vi "Calibrate_HH.vi"(3 "Deviceindex":i32) -> (0 "Returncode":i32, 1 "Status":string)   [LabVIEW 2009]
uses:
  hhlib.dll
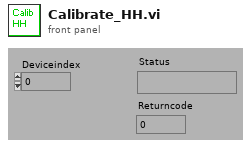
[diagram p1: front panel]
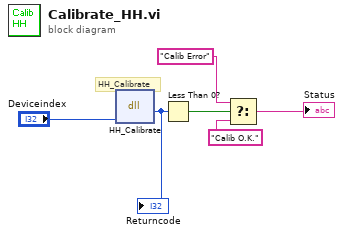
[diagram p0: block diagram]
diagram:
  # "HH_Calibrate"
  n1 = dll-call lib="C:/Programme/Anwendungen/DAQLinescan_HH/hhlib.dll" fn="HH_Calibrate"("devidx"="Deviceindex") -> (w4:i32)  [unwired: 4 in, 2 out]
  "Returncode" <- w4
  n2 = Less Than 0?(x=w4) -> (x < 0?=w2:bool)
  n3 = Select(t="Calib Error", s=w2, f="Calib O.K.") -> (s? t:f=→"Status":string)
